vi "VectorNav-ReadYPR.vi"() -> ()   [LabVIEW 2010]
uses:
  <vilib>/Instr/_visa.llb/VISA Configure Serial Port (Instr).vi
panel:
  in  "y":bool
  in  "VISA resource name":refnum<visa-resource-name>
  in  "stop":bool
  out "Roll":dbl
  out "Pitch":dbl
  out "Heading":dbl
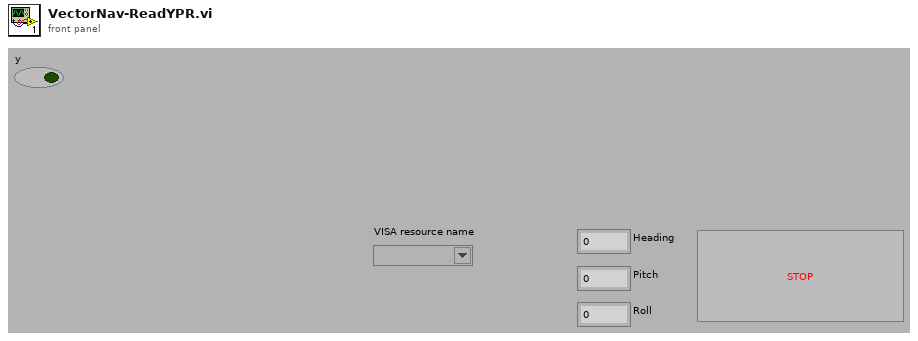
[diagram p1: front panel]
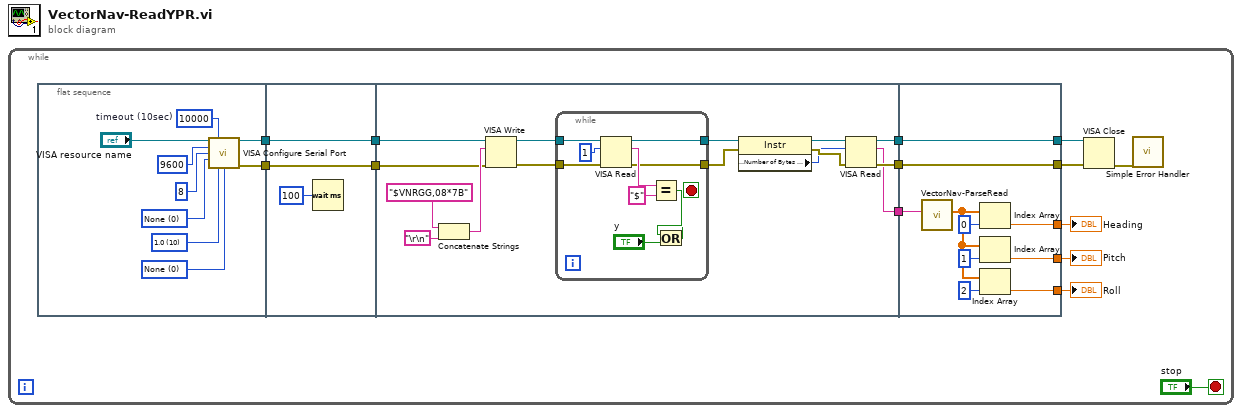
[diagram p0: block diagram]
diagram:
  n1 = while {
    stop <- "stop" stop-if-true
    n2 = flat-sequence {
      tunnel: [w16] -> w14
      tunnel: [w17] -> w13
      tunnel: w14 -> [w25]
      tunnel: w13 -> [w24]
      tunnel: [w25] -> w11
      tunnel: [w24] -> w12
      tunnel: [w34] -> w10
      tunnel: [w33] -> w9
      tunnel: [w32] -> w8
      tunnel: w12 -> [w28]
      tunnel: w11 -> [w27]
      tunnel: [w60] -> w5
      tunnel: [w61] -> w6
      tunnel: w10 -> [w61]
      tunnel: w9 -> [w60]
      tunnel: w8 -> [w59]
      tunnel: [w58] -> w4
      tunnel: [w54] -> w3
      tunnel: [w53] -> w2
      frame #0 {
        w19 = u16 0 items=["None"=0, "XON/XOFF"=1, "RTS/CTS"=2, "DTR/DSR"=4] ("flow control")
        w20 = u16 10 items=["1.0"=10, "1.5"=15, "2.0"=20] ("stop bits")
        w22 = u16 0 items=["None", "Odd", "Even", "Mark", "Space"] ("parity")
        w21 = u32 10000  # timeout (10sec)
        n3 = call-poly "VISA Configure Serial Port"("VISA resource name"="VISA resource name", "timeout (10sec)"=w21, "baud rate (9600)"=u32 9600 ("baud rate"), "data bits (8)"=u16 8 ("data bits"), "parity (0:none)"=w22, "stop bits (10: 1 bit)"=w20, "flow control (0:none)"=w19) -> ("VISA resource name out"=w17:refnum<visa-resource-name>, "error out"=w16:errorcluster)  [unwired: 2 in, 5 out]
      }
      frame #1 {
        n4 = Wait (ms)(milliseconds to wait=u32 100) -> ()  [unwired: 1 out]
      }
      frame #2 {
        n5 = Concatenate Strings("$VNRGG,08*7B" ("string"), "\r\n") -> (w29:string)
        n6 = VISA Write(VISA resource name=w28, write buffer=w29, error in (no error)=w27) -> (VISA resource name out=w36:refnum<visa-resource-name>, error out=w35:errorcluster)  [unwired: 1 out]
        n7 = while {
          tunnel: [w48] -> w37
          tunnel: [w47] -> w38
          tunnel: w36 -> [w46]
          tunnel: w35 -> [w45]
          stop <- w42 stop-if-true
          n8 = VISA Read(VISA resource name=w46, byte count=u32 1, error in (no error)=w45) -> (VISA resource name out=w48:refnum<visa-resource-name>, read buffer=w50:string, error out=w47:errorcluster)  [unwired: 1 out]
          n9 = Equal?(x=w50, y="$") -> (x = y?=w43:bool)
          n10 = Or(x=w43, y="y") -> (x .or. y?=w42:bool)
        }
        n11 = property class="Instr"(reference=w37, error in=w38) -> (reference out=w40:refnum<visa-resource-name>, error out=w41:errorcluster, "Serial Settings:Number of Bytes at Serial Port"=w39:u32)
        n12 = VISA Read(VISA resource name=w40, byte count=w39, error in (no error)=w41) -> (VISA resource name out=w34:refnum<visa-resource-name>, read buffer=w32:string, error out=w33:errorcluster)  [unwired: 1 out]
      }
      frame #3 {
        n13 = call "VectorNav-ParseRead.vi"("Input String"=w59) -> ("Output Array"=w57:dbl[])  [unwired: 10 in]
        n14 = Index Array(array=w57, index=0) -> (element=w58:dbl)
        n15 = Index Array(array=w57, index=1) -> (element=w54:dbl)
        n16 = Index Array(array=w57, index=2) -> (element=w53:dbl)
      }
    }
    n17 = VISA Close(VISA resource name=w6, error in (no error)=w5) -> (error out=w7:errorcluster)
    n18 = call <vilib>:"Simple Error Handler.vi"("error in (no error)"=w7) -> ()  [unwired: 1 in, 8 out]
    "Heading" <- w4
    "Pitch" <- w3
    "Roll" <- w2
  }
